vi "WILT Number of Button Presses.vi"(10 "Station Number":i32, 11 "Station Test State In":T1) -> (3 "Number of ON/OFF Cycles":i32=1)   [LabVIEW 2016]
uses:
  Type Definitions/WILT Station Test State Cluster.ctl
  Type Definitions/WILT Dryer Test State.ctl
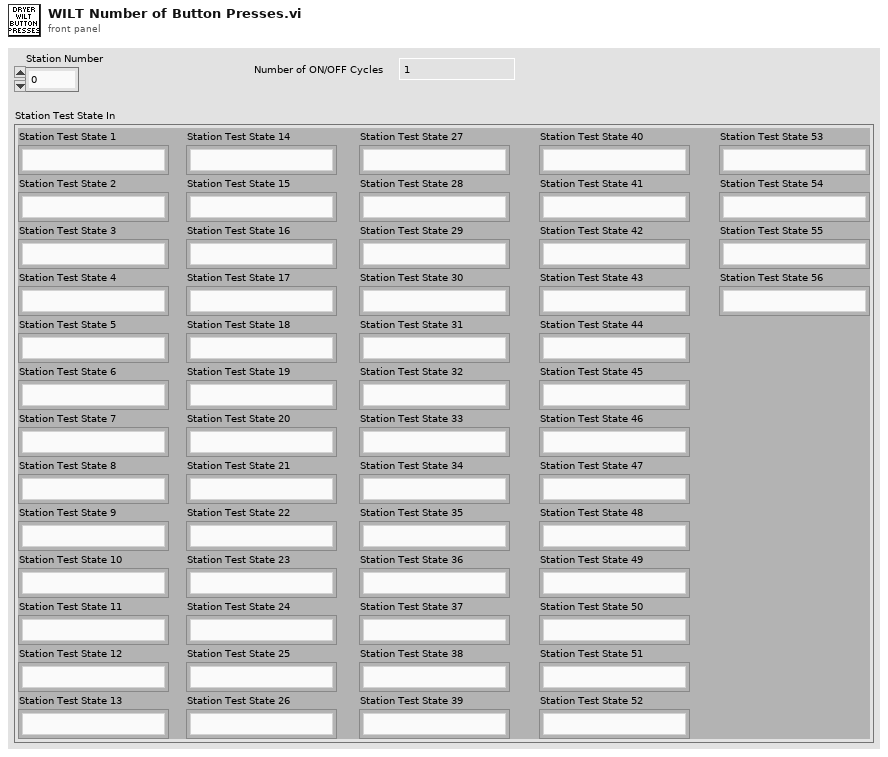
[diagram p1: front panel]
types:
  T1 = typedef "WILT Station Test State Cluster.ctl" = cluster{"Station Test State 1":T2, "Station Test State 2":T2, "Station Test State 3":T2, "Station Test State 4":T2, "Station Test State 5":T2, "Station Test State 6":T2, "Station Test State 7":T2, "Station Test State 8":T2, "Station Test State 9":T2, "Station Test State 10":T2, "Station Test State 11":T2, "Station Test State 12":T2, "Station Test State 13":T2, "Station Test State 14":T2, "Station Test State 15":T2, "Station Test State 16":T2, "Station Test State 17":T2, "Station Test State 18":T2, "Station Test State 19":T2, "Station Test State 20":T2, "Station Test State 21":T2, "Station Test State 22":T2, "Station Test State 23":T2, "Station Test State 24":T2, "Station Test State 25":T2, "Station Test State 26":T2, "Station Test State 27":T2, "Station Test State 28":T2, "Station Test State 29":T2, "Station Test State 30":T2, "Station Test State 31":T2, "Station Test State 32":T2, "Station Test State 33":T2, "Station Test State 34":T2, "Station Test State 35":T2, "Station Test State 36":T2, "Station Test State 37":T2, "Station Test State 38":T2, "Station Test State 39":T2, "Station Test State 40":T2, "Station Test State 41":T2, "Station Test State 42":T2, "Station Test State 43":T2, "Station Test State 44":T2, "Station Test State 45":T2, "Station Test State 46":T2, "Station Test State 47":T2, "Station Test State 48":T2, "Station Test State 49":T2, "Station Test State 50":T2, "Station Test State 51":T2, "Station Test State 52":T2, "Station Test State 53":T2, "Station Test State 54":T2, "Station Test State 55":T2, "Station Test State 56":T2}
  T2 = typedef "WILT Dryer Test State.ctl" = enum16{"No Serial Number", "Waiting for Dryer To Start", "Drying Clothes", "Water Injection 1 (On)", "Water Injection 1 Timer", "Water Injection 1 (Off)", "Pause Dryer", "Sending Start Stop CMD", "Pause Dryer 2", "Sending Start Stop CMD 2", "Drying Clothes 2", "Water Injection 2 (On)", "Water Injection 2 Timer", "Water Injection 2 (Off)", "Drying Clothes 3", "Cooling Down", "Sending Start Stop CMD 3", "Increment Cycle"}
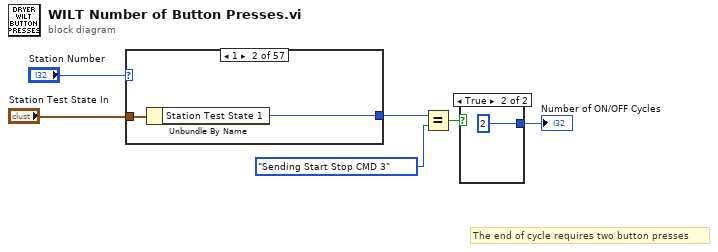
[diagram p0: block diagram]
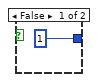
[diagram p2: hidden frame]
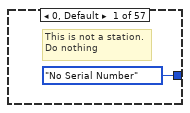
[diagram p3: hidden frame]
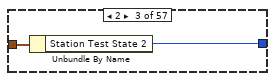
[diagram p4: hidden frame]
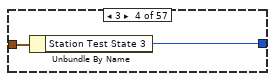
[diagram p5: hidden frame]
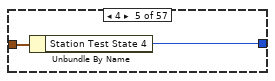
[diagram p6: hidden frame]
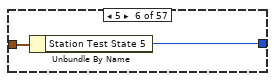
[diagram p7: hidden frame]
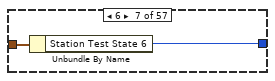
[diagram p8: hidden frame]
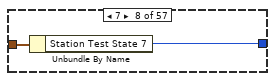
[diagram p9: hidden frame]
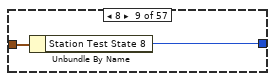
[diagram p10: hidden frame]
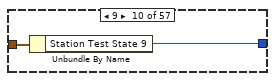
[diagram p11: hidden frame]
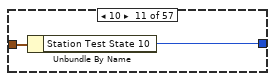
[diagram p12: hidden frame]
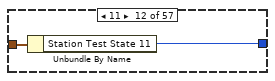
[diagram p13: hidden frame]
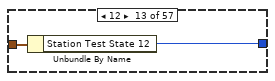
[diagram p14: hidden frame]
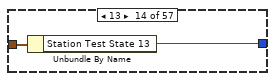
[diagram p15: hidden frame]
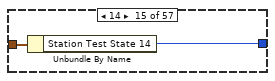
[diagram p16: hidden frame]
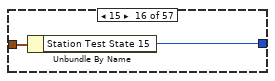
[diagram p17: hidden frame]
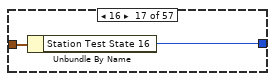
[diagram p18: hidden frame]
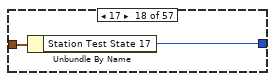
[diagram p19: hidden frame]
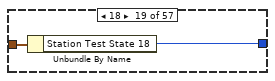
[diagram p20: hidden frame]
diagram:
  # "The end of cycle requires two button presses"
  n1 = case shown="1" "Station Number" {
    tunnel: "Station Test State In" -> [_ w9 w11 w13 w15 w17 w19 w21 w23 w25 w27 w29 w31 w33 w35 w37 w39 w41 w43 w45 w47 w49 w51 w53 w55 w57 w59 w61 w63 w65 w67 w69 w71 w73 w75 w77 w79 w81 w83 w85 w87 w89 w91 w93 w95 w97 w99 w101 w103 w105 w107 w109 w111 w113 w115 w117 w119]
    tunnel: [WILT_Dryer_Test_State."No Serial Number" ("Station Test State 56") w8 w10 w12 w14 w16 w18 w20 w22 w24 w26 w28 w30 w32 w34 w36 w38 w40 w42 w44 w46 w48 w50 w52 w54 w56 w58 w60 w62 w64 w66 w68 w70 w72 w74 w76 w78 w80 w82 w84 w86 w88 w90 w92 w94 w96 w98 w100 w102 w104 w106 w108 w110 w112 w114 w116 w118] -> w4
    frame 0, Default {
      # "This is not a station.\nDo nothing"
    }
    frame 1 {
      n2 = Unbundle By Name(w9) -> ("Station Test State 1"=w8:T2)
    }
    frame 2 {
      n3 = Unbundle By Name(w11) -> ("Station Test State 2"=w10:T2)
    }
    frame 3 {
      n4 = Unbundle By Name(w13) -> ("Station Test State 3"=w12:T2)
    }
    frame 4 {
      n5 = Unbundle By Name(w15) -> ("Station Test State 4"=w14:T2)
    }
    frame 5 {
      n6 = Unbundle By Name(w17) -> ("Station Test State 5"=w16:T2)
    }
    frame 6 {
      n7 = Unbundle By Name(w19) -> ("Station Test State 6"=w18:T2)
    }
    frame 7 {
      n8 = Unbundle By Name(w21) -> ("Station Test State 7"=w20:T2)
    }
    frame 8 {
      n9 = Unbundle By Name(w23) -> ("Station Test State 8"=w22:T2)
    }
    frame 9 {
      n10 = Unbundle By Name(w25) -> ("Station Test State 9"=w24:T2)
    }
    frame 10 {
      n11 = Unbundle By Name(w27) -> ("Station Test State 10"=w26:T2)
    }
    frame 11 {
      n12 = Unbundle By Name(w29) -> ("Station Test State 11"=w28:T2)
    }
    frame 12 {
      n13 = Unbundle By Name(w31) -> ("Station Test State 12"=w30:T2)
    }
    frame 13 {
      n14 = Unbundle By Name(w33) -> ("Station Test State 13"=w32:T2)
    }
    frame 14 {
      n15 = Unbundle By Name(w35) -> ("Station Test State 14"=w34:T2)
    }
    frame 15 {
      n16 = Unbundle By Name(w37) -> ("Station Test State 15"=w36:T2)
    }
    frame 16 {
      n17 = Unbundle By Name(w39) -> ("Station Test State 16"=w38:T2)
    }
    frame 17 {
      n18 = Unbundle By Name(w41) -> ("Station Test State 17"=w40:T2)
    }
    frame 18 {
      n19 = Unbundle By Name(w43) -> ("Station Test State 18"=w42:T2)
    }
    frame 19 {
      n20 = Unbundle By Name(w45) -> ("Station Test State 19"=w44:T2)
    }
    frame 20 {
      n21 = Unbundle By Name(w47) -> ("Station Test State 20"=w46:T2)
    }
    frame 21 {
      n22 = Unbundle By Name(w49) -> ("Station Test State 21"=w48:T2)
    }
    frame 22 {
      n23 = Unbundle By Name(w51) -> ("Station Test State 22"=w50:T2)
    }
    frame 23 {
      n24 = Unbundle By Name(w53) -> ("Station Test State 23"=w52:T2)
    }
    frame 24 {
      n25 = Unbundle By Name(w55) -> ("Station Test State 24"=w54:T2)
    }
    frame 25 {
      n26 = Unbundle By Name(w57) -> ("Station Test State 25"=w56:T2)
    }
    frame 26 {
      n27 = Unbundle By Name(w59) -> ("Station Test State 26"=w58:T2)
    }
    frame 27 {
      n28 = Unbundle By Name(w61) -> ("Station Test State 27"=w60:T2)
    }
    frame 28 {
      n29 = Unbundle By Name(w63) -> ("Station Test State 28"=w62:T2)
    }
    frame 29 {
      n30 = Unbundle By Name(w65) -> ("Station Test State 29"=w64:T2)
    }
    frame 30 {
      n31 = Unbundle By Name(w67) -> ("Station Test State 30"=w66:T2)
    }
    frame 31 {
      n32 = Unbundle By Name(w69) -> ("Station Test State 31"=w68:T2)
    }
    frame 32 {
      n33 = Unbundle By Name(w71) -> ("Station Test State 32"=w70:T2)
    }
    frame 33 {
      n34 = Unbundle By Name(w73) -> ("Station Test State 33"=w72:T2)
    }
    frame 34 {
      n35 = Unbundle By Name(w75) -> ("Station Test State 34"=w74:T2)
    }
    frame 35 {
      n36 = Unbundle By Name(w77) -> ("Station Test State 35"=w76:T2)
    }
    frame 36 {
      n37 = Unbundle By Name(w79) -> ("Station Test State 36"=w78:T2)
    }
    frame 37 {
      n38 = Unbundle By Name(w81) -> ("Station Test State 37"=w80:T2)
    }
    frame 38 {
      n39 = Unbundle By Name(w83) -> ("Station Test State 38"=w82:T2)
    }
    frame 39 {
      n40 = Unbundle By Name(w85) -> ("Station Test State 39"=w84:T2)
    }
    frame 40 {
      n41 = Unbundle By Name(w87) -> ("Station Test State 40"=w86:T2)
    }
    frame 41 {
      n42 = Unbundle By Name(w89) -> ("Station Test State 41"=w88:T2)
    }
    frame 42 {
      n43 = Unbundle By Name(w91) -> ("Station Test State 42"=w90:T2)
    }
    frame 43 {
      n44 = Unbundle By Name(w93) -> ("Station Test State 43"=w92:T2)
    }
    frame 44 {
      n45 = Unbundle By Name(w95) -> ("Station Test State 44"=w94:T2)
    }
    frame 45 {
      n46 = Unbundle By Name(w97) -> ("Station Test State 45"=w96:T2)
    }
    frame 46 {
      n47 = Unbundle By Name(w99) -> ("Station Test State 46"=w98:T2)
    }
    frame 47 {
      n48 = Unbundle By Name(w101) -> ("Station Test State 47"=w100:T2)
    }
    frame 48 {
      n49 = Unbundle By Name(w103) -> ("Station Test State 48"=w102:T2)
    }
    frame 49 {
      n50 = Unbundle By Name(w105) -> ("Station Test State 49"=w104:T2)
    }
    frame 50 {
      n51 = Unbundle By Name(w107) -> ("Station Test State 50"=w106:T2)
    }
    frame 51 {
      n52 = Unbundle By Name(w109) -> ("Station Test State 51"=w108:T2)
    }
    frame 52 {
      n53 = Unbundle By Name(w111) -> ("Station Test State 52"=w110:T2)
    }
    frame 53 {
      n54 = Unbundle By Name(w113) -> ("Station Test State 53"=w112:T2)
    }
    frame 54 {
      n55 = Unbundle By Name(w115) -> ("Station Test State 54"=w114:T2)
    }
    frame 55 {
      n56 = Unbundle By Name(w117) -> ("Station Test State 55"=w116:T2)
    }
    frame 56 {
      n57 = Unbundle By Name(w119) -> ("Station Test State 56"=w118:T2)
    }
  }
  n58 = Equal?(x=w4, y=WILT_Dryer_Test_State."Sending Start Stop CMD 3") -> (x = y?=w2:bool)
  n59 = case shown="True" w2 {
    tunnel: [1 2] -> w1
    frame False {
    }
    frame True {
    }
  }
  "Number of ON/OFF Cycles" <- w1
